vi "Get.vi"(8 "error in (no error)":errorcluster, 11 "Waveform Generator in":refnum<class "Waveform Generator.lvclass">) -> (0 "error out":errorcluster, 2 "Value":dbl, 3 "Waveform Generator out":refnum<class "Waveform Generator.lvclass">)   [LabVIEW 2015, in "Waveform Generator.lvclass"]
uses:
  Waveform Generator.lvclass
  Waveform Generator.lvclass/Waveform Generator.ctl
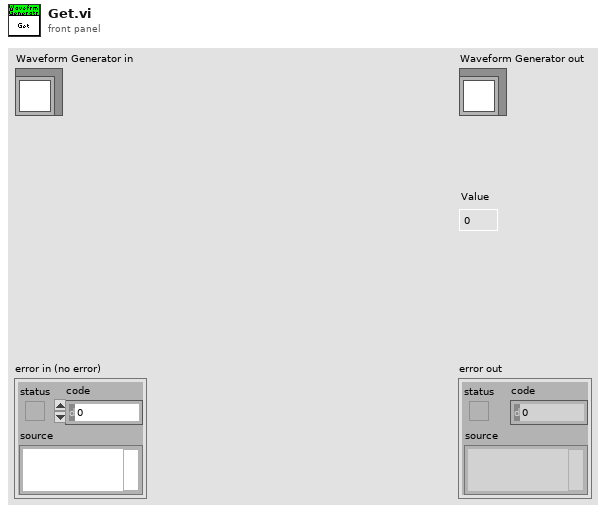
[diagram p1: front panel]
types:
  T1 = typedef "FAMT Typedefs.lvlib/Waveform Types.ctl" = enum16{"Sine", "Triangle", "Square", "Sawtooth", "Chirp", "Gaussian", "Trapezoid", "Constant"}
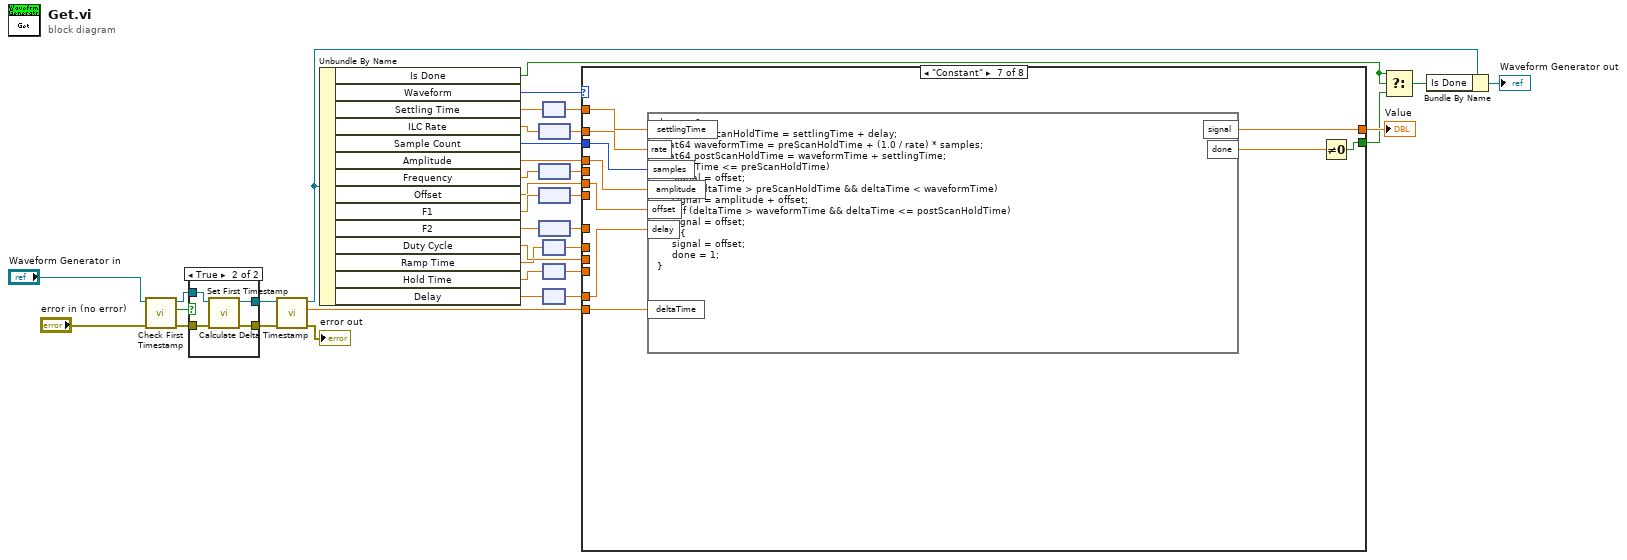
[diagram p0: block diagram]
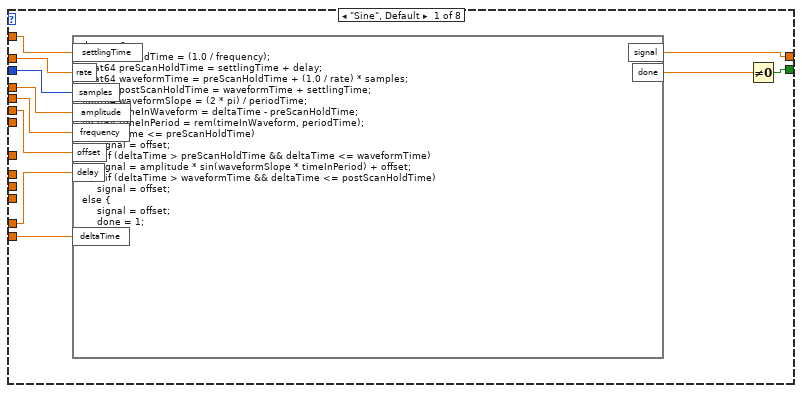
[diagram p2: hidden frame]
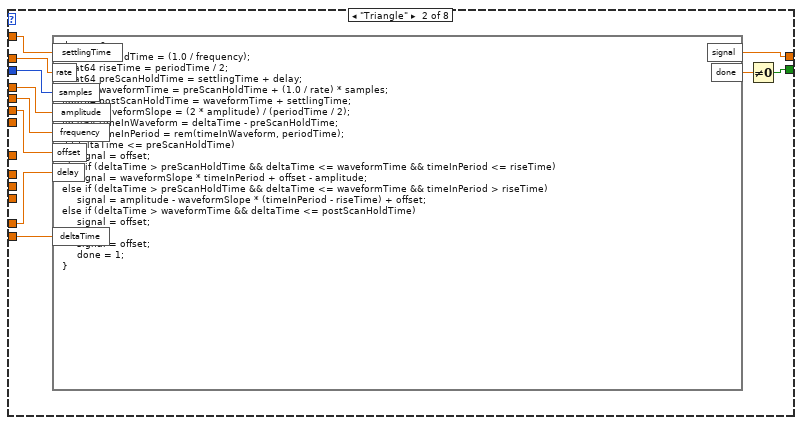
[diagram p3: hidden frame]
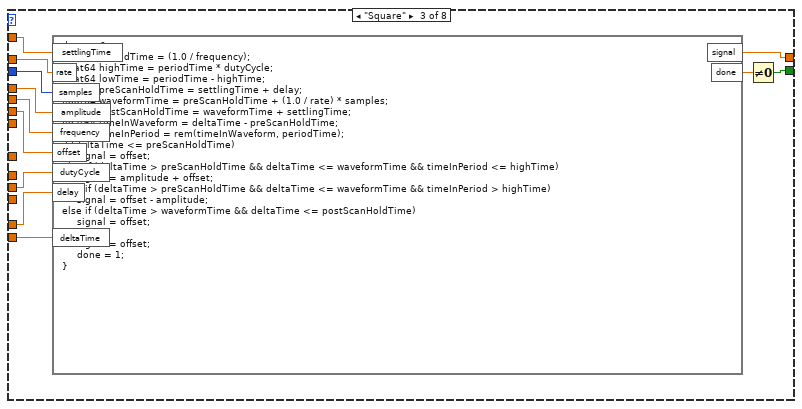
[diagram p4: hidden frame]
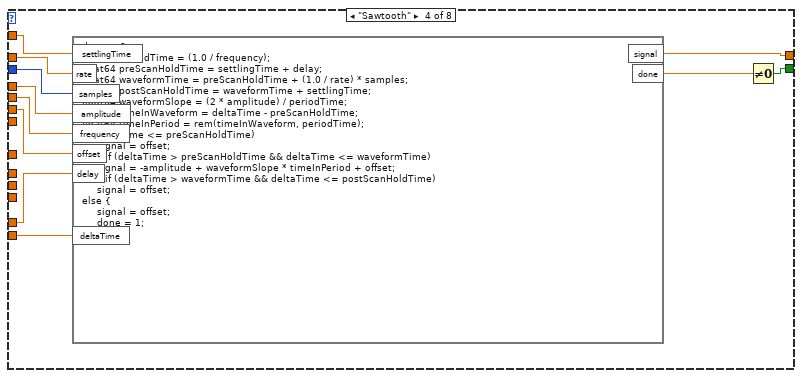
[diagram p5: hidden frame]
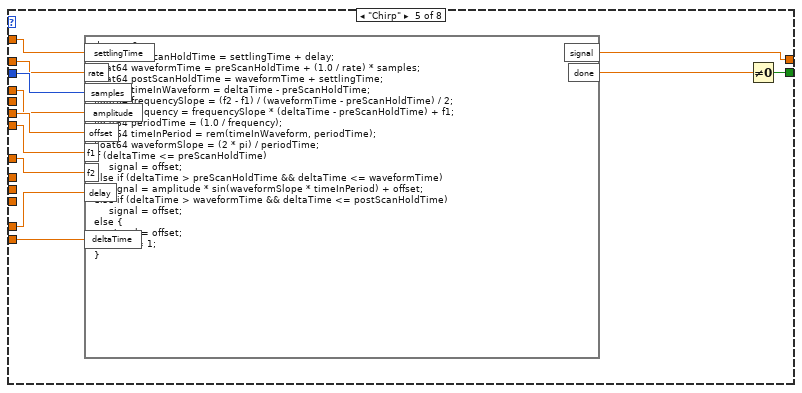
[diagram p6: hidden frame]
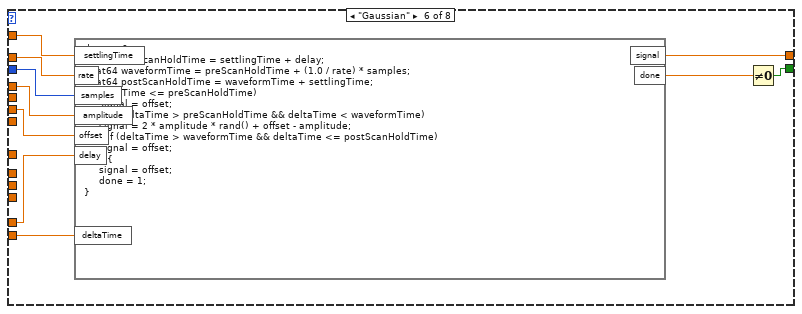
[diagram p7: hidden frame]
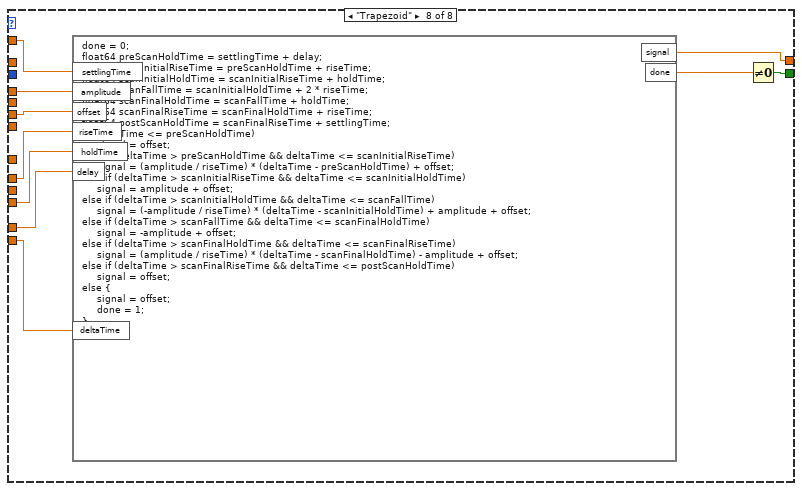
[diagram p8: hidden frame]
diagram:
  n1 = call "Check First Timestamp.vi"("error in (no error)"="error in (no error)", "Waveform Generator in"="Waveform Generator in") -> ("error out"=w34:errorcluster, "Is First"=w36:bool, "Waveform Generator out"=w35:refnum<class "Waveform Generator.lvclass">)  [unwired: 7 in]
  n2 = case shown="True" w36 {
    tunnel: w35 -> [w38 w42]
    tunnel: [w38 w41] -> w33
    tunnel: w34 -> [w37 w40]
    tunnel: [w37 w39] -> w32
    frame False {
    }
    frame True {
      n3 = call "Set First Timestamp.vi"("error in (no error)"=w40, "Waveform Generator in"=w42) -> ("error out"=w39:errorcluster, "Waveform Generator out"=w41:refnum<class "Waveform Generator.lvclass">)  [unwired: 8 in]
    }
  }
  n4 = call "Calculate Delta Timestamp.vi"("error in (no error)"=w32, "Waveform Generator in"=w33) -> ("error out"=→"error out":errorcluster, "Delta Timestamp"=w19:dbl, "Waveform Generator out"=w9:refnum<class "Waveform Generator.lvclass">)  [unwired: 7 in]
  n5 = Unbundle By Name(w9) -> ("Is Done"=w6:bool, "Waveform"=w17:T1, "Settling Time"=w30:dbl[unit], "ILC Rate"=w28:dbl[unit], "Sample Count"=w27:u32, "Amplitude"=w4:dbl, "Frequency"=w16:dbl[unit], "Offset"=w3:dbl, "F1"=w25:dbl[unit], "F2"=w23:dbl[unit], "Duty Cycle"=w14:dbl, "Ramp Time"=w13:dbl[unit], "Hold Time"=w12:dbl[unit], "Delay"=w2:dbl[unit])
  n6 = node(w28) -> (w26:dbl)
  n7 = node(w16) -> (w15:dbl)
  n8 = node(w25) -> (w24:dbl)
  n9 = node(w23) -> (w22:dbl)
  n10 = node(w30) -> (w29:dbl)
  n11 = node(w13) -> (w10:dbl)
  n12 = node(w12) -> (w11:dbl)
  n13 = node(w2) -> (w1:dbl)
  n14 = case shown="\"Constant\"" w17 {
    tunnel: [w46 w64 w68 w80 w91 w104 w114 w123] -> w31
    tunnel: w29 -> [w53 w57 w70 w87 w92 w109 w119 w129]
    tunnel: w27 -> [w51 w59 w72 w85 w94 w107 w117 _]
    tunnel: w26 -> [w52 w58 w71 w86 w93 w108 w118 _]
    tunnel: w4 -> [w50 w60 w73 w84 w95 w106 w116 w128]
    tunnel: w3 -> [w49 w62 w75 w82 w96 w101 w111 w127]
    tunnel: w24 -> [_ _ _ _ w97 _ _ _]
    tunnel: w22 -> [_ _ _ _ w98 _ _ _]
    tunnel: w19 -> [w47 w63 w69 w81 w99 w105 w115 w124]
    tunnel: w15 -> [w48 w61 w74 w83 _ _ _ _]
    tunnel: w14 -> [_ _ w76 _ _ _ _ _]
    tunnel: w11 -> [_ _ _ _ _ _ _ w126]
    tunnel: w10 -> [_ _ _ _ _ _ _ w125]
    tunnel: [w45 w55 w67 w78 w89 w102 w112 w121] -> w7
    tunnel: w1 -> [w43 w54 w65 w77 w88 w100 w110 w120]
    frame "Sine", Default {
      n15 = formula code="done = 0;\nfloat64 periodTime = (1.0 / frequency);\nfloat64 preScanHoldTime = settlingTime + delay;\nfloat64 waveformTime = preScanHoldTime + (1.0 / rate) * samples;\nfloat64 postScanHoldTime = waveformTime + settlingTime;\nfloat64 waveformSlope = (2 * pi) / periodTime;\nfloat64 timeInWaveform = deltaTime - preScanHoldTime;\nfloat64 timeInPeriod = rem(timeInWaveform, periodTime);\nif (deltaTime <= preScanHoldTime)\n     signal = offset;\nelse if (deltaTime > preScanHoldTime && deltaTime <= waveformTime)\n     signal = amplitude * sin(waveformSlope * timeInPeriod) + offset;\nelse if (deltaTime > waveformTime && deltaTime <= postScanHoldTime)\n     signal = offset;\nelse {\n     signal = offset;\n     done = 1;\n}"("rate"=w52, "settlingTime"=w53, "samples"=w51, "amplitude"=w50, "frequency"=w48, "offset"=w49, "deltaTime"=w47, "delay"=w43) -> ("signal"=w46:dbl, "done"=w44:dbl)
      n16 = Not Equal To 0?(x=w44) -> (x != 0?=w45:bool)
    }
    frame "Triangle" {
      n17 = formula code="done = 0;\nfloat64 periodTime = (1.0 / frequency);\nfloat64 riseTime = periodTime / 2;\nfloat64 preScanHoldTime = settlingTime + delay;\nfloat64 waveformTime = preScanHoldTime + (1.0 / rate) * samples;\nfloat64 postScanHoldTime = waveformTime + settlingTime;\nfloat64 waveformSlope = (2 * amplitude) / (periodTime / 2);\nfloat64 timeInWaveform = deltaTime - preScanHoldTime;\nfloat64 timeInPeriod = rem(timeInWaveform, periodTime);\nif (deltaTime <= preScanHoldTime)\n     signal = offset;\nelse if (deltaTime > preScanHoldTime && deltaTime <= waveformTime && timeInPeriod <= riseTime)\n     signal = waveformSlope * timeInPeriod + offset - amplitude;\nelse if (deltaTime > preScanHoldTime && deltaTime <= waveformTime && timeInPeriod > riseTime)\n     signal = amplitude - waveformSlope * (timeInPeriod - riseTime) + offset;\nelse if (deltaTime > waveformTime && deltaTime <= postScanHoldTime)\n     signal = offset;\nelse {\n     signal = offset;\n     done = 1;\n}"("rate"=w58, "settlingTime"=w57, "samples"=w59, "amplitude"=w60, "frequency"=w61, "offset"=w62, "deltaTime"=w63, "delay"=w54) -> ("signal"=w64:dbl, "done"=w56:dbl)
      n18 = Not Equal To 0?(x=w56) -> (x != 0?=w55:bool)
    }
    frame "Square" {
      n19 = formula code="done = 0;\nfloat64 periodTime = (1.0 / frequency);\nfloat64 highTime = periodTime * dutyCycle;\nfloat64 lowTime = periodTime - highTime;\nfloat64 preScanHoldTime = settlingTime + delay;\nfloat64 waveformTime = preScanHoldTime + (1.0 / rate) * samples;\nfloat64 postScanHoldTime = waveformTime + settlingTime;\nfloat64 timeInWaveform = deltaTime - preScanHoldTime;\nfloat64 timeInPeriod = rem(timeInWaveform, periodTime);\nif (deltaTime <= preScanHoldTime)\n     signal = offset;\nelse if (deltaTime > preScanHoldTime && deltaTime <= waveformTime && timeInPeriod <= highTime)\n     signal = amplitude + offset;\nelse if (deltaTime > preScanHoldTime && deltaTime <= waveformTime && timeInPeriod > highTime)\n     signal = offset - amplitude;\nelse if (deltaTime > waveformTime && deltaTime <= postScanHoldTime)\n     signal = offset;\nelse {\n     signal = offset;\n     done = 1;\n}"("rate"=w71, "settlingTime"=w70, "samples"=w72, "amplitude"=w73, "frequency"=w74, "offset"=w75, "deltaTime"=w69, "dutyCycle"=w76, "delay"=w65) -> ("signal"=w68:dbl, "done"=w66:dbl)
      n20 = Not Equal To 0?(x=w66) -> (x != 0?=w67:bool)
    }
    frame "Sawtooth" {
      n21 = formula code="done = 0;\nfloat64 periodTime = (1.0 / frequency);\nfloat64 preScanHoldTime = settlingTime + delay;\nfloat64 waveformTime = preScanHoldTime + (1.0 / rate) * samples;\nfloat64 postScanHoldTime = waveformTime + settlingTime;\nfloat64 waveformSlope = (2 * amplitude) / periodTime;\nfloat64 timeInWaveform = deltaTime - preScanHoldTime;\nfloat64 timeInPeriod = rem(timeInWaveform, periodTime);\nif (deltaTime <= preScanHoldTime)\n     signal = offset;\nelse if (deltaTime > preScanHoldTime && deltaTime <= waveformTime)\n     signal = -amplitude + waveformSlope * timeInPeriod + offset;\nelse if (deltaTime > waveformTime && deltaTime <= postScanHoldTime)\n     signal = offset;\nelse {\n     signal = offset;\n     done = 1;\n}"("rate"=w86, "settlingTime"=w87, "samples"=w85, "amplitude"=w84, "frequency"=w83, "offset"=w82, "deltaTime"=w81, "delay"=w77) -> ("signal"=w80:dbl, "done"=w79:dbl)
      n22 = Not Equal To 0?(x=w79) -> (x != 0?=w78:bool)
    }
    frame "Chirp" {
      n23 = formula code="done = 0;\nfloat64 preScanHoldTime = settlingTime + delay;\nfloat64 waveformTime = preScanHoldTime + (1.0 / rate) * samples;\nfloat64 postScanHoldTime = waveformTime + settlingTime;\nfloat64 timeInWaveform = deltaTime - preScanHoldTime;\nfloat64 frequencySlope = (f2 - f1) / (waveformTime - preScanHoldTime) / 2;\nfloat64 frequency = frequencySlope * (deltaTime - preScanHoldTime) + f1;\nfloat64 periodTime = (1.0 / frequency);\nfloat64 timeInPeriod = rem(timeInWaveform, periodTime);\nfloat64 waveformSlope = (2 * pi) / periodTime;\nif (deltaTime <= preScanHoldTime)\n     signal = offset;\nelse if (deltaTime > preScanHoldTime && deltaTime <= waveformTime)\n     signal = amplitude * sin(waveformSlope * timeInPeriod) + offset;\nelse if (deltaTime > waveformTime && deltaTime <= postScanHoldTime)\n     signal = offset;\nelse {\n     signal = offset;\n     done = 1;\n}"("rate"=w93, "settlingTime"=w92, "samples"=w94, "amplitude"=w95, "offset"=w96, "deltaTime"=w99, "f1"=w97, "f2"=w98, "delay"=w88) -> ("signal"=w91:dbl, "done"=w90:dbl)
      n24 = Not Equal To 0?(x=w90) -> (x != 0?=w89:bool)
    }
    frame "Gaussian" {
      n25 = formula code="done = 0;\nfloat64 preScanHoldTime = settlingTime + delay;\nfloat64 waveformTime = preScanHoldTime + (1.0 / rate) * samples;\nfloat64 postScanHoldTime = waveformTime + settlingTime;\nif (deltaTime <= preScanHoldTime)\n     signal = offset;\nelse if (deltaTime > preScanHoldTime && deltaTime < waveformTime)\n     signal = 2 * amplitude * rand() + offset - amplitude;\nelse if (deltaTime > waveformTime && deltaTime <= postScanHoldTime)\n     signal = offset;\nelse {\n     signal = offset;\n     done = 1;\n}"("settlingTime"=w109, "amplitude"=w106, "offset"=w101, "deltaTime"=w105, "rate"=w108, "samples"=w107, "delay"=w100) -> ("signal"=w104:dbl, "done"=w103:dbl)
      n26 = Not Equal To 0?(x=w103) -> (x != 0?=w102:bool)
    }
    frame "Constant" {
      n27 = formula code="done = 0;\nfloat64 preScanHoldTime = settlingTime + delay;\nfloat64 waveformTime = preScanHoldTime + (1.0 / rate) * samples;\nfloat64 postScanHoldTime = waveformTime + settlingTime;\nif (deltaTime <= preScanHoldTime)\n     signal = offset;\nelse if (deltaTime > preScanHoldTime && deltaTime < waveformTime)\n     signal = amplitude + offset;\nelse if (deltaTime > waveformTime && deltaTime <= postScanHoldTime)\n     signal = offset;\nelse {\n     signal = offset;\n     done = 1;\n}"("settlingTime"=w119, "amplitude"=w116, "offset"=w111, "deltaTime"=w115, "rate"=w118, "samples"=w117, "delay"=w110) -> ("signal"=w114:dbl, "done"=w113:dbl)
      n28 = Not Equal To 0?(x=w113) -> (x != 0?=w112:bool)
    }
    frame "Trapezoid" {
      n29 = formula code="done = 0;\nfloat64 preScanHoldTime = settlingTime + delay;\nfloat64 scanInitialRiseTime = preScanHoldTime + riseTime;\nfloat64 scanInitialHoldTime = scanInitialRiseTime + holdTime;\nfloat64 scanFallTime = scanInitialHoldTime + 2 * riseTime;\nfloat64 scanFinalHoldTime = scanFallTime + holdTime;\nfloat64 scanFinalRiseTime = scanFinalHoldTime + riseTime;\nfloat64 postScanHoldTime = scanFinalRiseTime + settlingTime;\nif (deltaTime <= preScanHoldTime)\n     signal = offset;\nelse if (deltaTime > preScanHoldTime && deltaTime <= scanInitialRiseTime)\n     signal = (amplitude / riseTime) * (deltaTime - preScanHoldTime) + offset;\nelse if (deltaTime > scanInitialRiseTime && deltaTime <= scanInitialHoldTime)\n     signal = amplitude + offset;\nelse if (deltaTime > scanInitialHoldTime && deltaTime <= scanFallTime)\n     signal = (-amplitude / riseTime) * (deltaTime - scanInitialHoldTime) + amplitude + offset;\nelse if (deltaTime > scanFallTime && deltaTime <= scanFinalHoldTime)\n     signal = -amplitude + offset;\nelse if (deltaTime > scanFinalHoldTime && deltaTime <= scanFinalRiseTime)\n     signal = (amplitude / riseTime) * (deltaTime - scanFinalHoldTime) - amplitude + offset;\nelse if (deltaTime > scanFinalRiseTime && deltaTime <= postScanHoldTime)\n     signal = offset;\nelse {\n     signal = offset;\n     done = 1;\n}"("deltaTime"=w124, "riseTime"=w125, "holdTime"=w126, "amplitude"=w128, "offset"=w127, "settlingTime"=w129, "delay"=w120) -> ("signal"=w123:dbl, "done"=w122:dbl)
      n30 = Not Equal To 0?(x=w122) -> (x != 0?=w121:bool)
    }
  }
  "Value" <- w31
  n31 = Select(t=w6, s=w6, f=w7) -> (s? t:f=w5:bool)
  n32 = Bundle By Name(cluster=w9, "Is Done"=w5) -> (→"Waveform Generator out":refnum<class "Waveform Generator.lvclass">)
